vi "TSP-Link State.vi"(8 "error in (no error)":errorcluster, 11 "VISA resource name":refnum<visa-resource-name>) -> (0 "error out":errorcluster, 2 "State":string, 3 "VISA resource name out":refnum<visa-resource-name>, 4 "Command String":string)   [LabVIEW 2013, in "Keithley 2600 Series.lvlib"]
doc: "This VI returns the TSP-Link on-line state.\n\n<b>Functions and Attributes Used</b>\ntsplink.state\n\nNote:\nTSP-Link feature is not supported with Keithley 2604B, 2614B, 2634B."
uses:
  Keithley 2600 Series.lvlib
  Private/GlobalVariables.vi
panel:
  # "(c) 2008 Keithley Instruments, Inc.  ALL RIGHTS RESERVED."
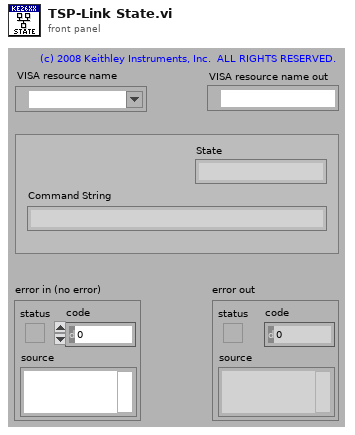
[diagram p1: front panel]
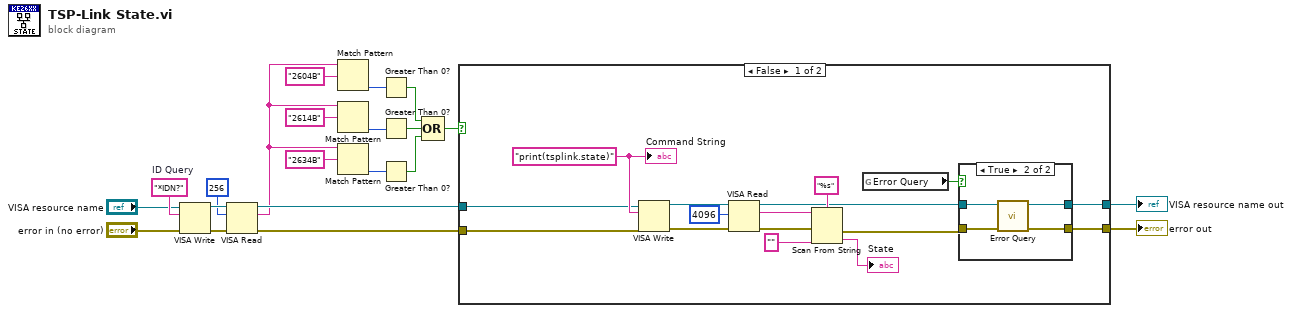
[diagram p0: block diagram]
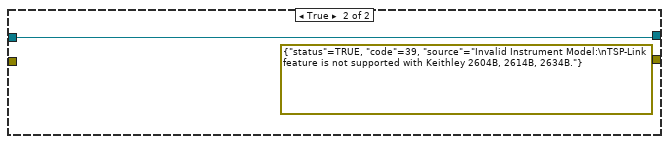
[diagram p3: hidden frame]
diagram:
  w16 = "*IDN?"  # ID Query
  n1 = VISA Write(VISA resource name="VISA resource name", write buffer=w16, error in (no error)="error in (no error)") -> (VISA resource name out=w19:refnum<visa-resource-name>, error out=w18:errorcluster)  [unwired: 1 out]
  n2 = VISA Read(VISA resource name=w19, byte count=u32 256, error in (no error)=w18) -> (VISA resource name out=w15:refnum<visa-resource-name>, read buffer=w1:string, error out=w14:errorcluster)  [unwired: 1 out]
  n3 = Match Pattern(string=w1, regular expression="2604B" ("y")) -> (offset past match=w8:i32)  [unwired: 1 in, 3 out]
  n4 = Match Pattern(string=w1, regular expression="2614B" ("y")) -> (offset past match=w7:i32)  [unwired: 1 in, 3 out]
  n5 = Match Pattern(string=w1, regular expression="2634B" ("y")) -> (offset past match=w6:i32)  [unwired: 1 in, 3 out]
  n6 = Greater Than 0?(x=w8) -> (x > 0?=w5:bool)
  n7 = Greater Than 0?(x=w7) -> (x > 0?=w4:bool)
  n8 = Greater Than 0?(x=w6) -> (x > 0?=w3:bool)
  n9 = Compound Arithmetic op=OR(w5, w4, w3) -> (w2:bool)
  n10 = case shown="False" w2 {
    tunnel: [w25 w45] -> w21
    tunnel: [w24 errorcluster {"status"=TRUE, "code"=39, "source"="Invalid Instrument Model:\nTSP-Link feature is not supported with Keithley 2604B, 2614B, 2634B."} ("error out")] -> w20
    tunnel: w15 -> [w23 w45]
    tunnel: w14 -> [w22 _]
    frame False {
      w29 = "print(tsplink.state)" ("command")
      n11 = VISA Write(VISA resource name=w23, write buffer=w29, error in (no error)=w22) -> (VISA resource name out=w37:refnum<visa-resource-name>, error out=w36:errorcluster)  [unwired: 1 out]
      n12 = VISA Read(VISA resource name=w37, byte count=u32 4096, error in (no error)=w36) -> (VISA resource name out=w27:refnum<visa-resource-name>, read buffer=w34:string, error out=w32:errorcluster)  [unwired: 1 out]
      n13 = Scan From String(format string="%s", input string=w34, error in=w32, default 1="" ("default value 1")) -> (error out=w26:errorcluster, output 1=→"State":string)  [unwired: 1 in, 2 out]
      n14 = global read "GlobalVariables.vi" "Error Query"() -> (w28:bool)
      n15 = case shown="True" w28 {
        tunnel: w27 -> [w39 w43]
        tunnel: w26 -> [w38 w42]
        tunnel: [w39 w41] -> w25
        tunnel: [w38 w40] -> w24
        frame False {
        }
        frame True {
          n16 = call "Error Query.vi"("error in (no error)"=w42, "VISA resource name"=w43) -> ("error out"=w40:errorcluster, "VISA resource name out"=w41:refnum<visa-resource-name>)  [unwired: 8 out]
        }
      }
      "Command String" <- w29
    }
    frame True {
    }
  }
  "VISA resource name out" <- w21
  "error out" <- w20
